vi "Module A.vi"(8 "Error In":errorcluster) -> (0 "Error Out":errorcluster)   [LabVIEW 2024]
panel:
  in  "Stop":bool
  out "Elapsed Time":dbl format="%.3f seconds"
  out "Loop iteration":i32
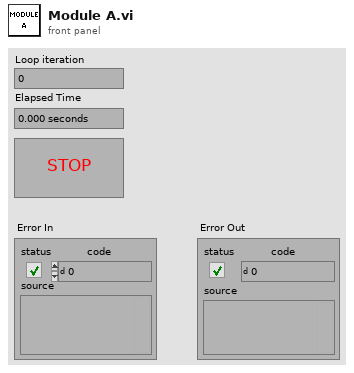
[diagram p1: front panel]
types:
  T1 = enum32{"Invalid", "Standard", "Closed", "Hidden", "Minimized", "Maximized"}
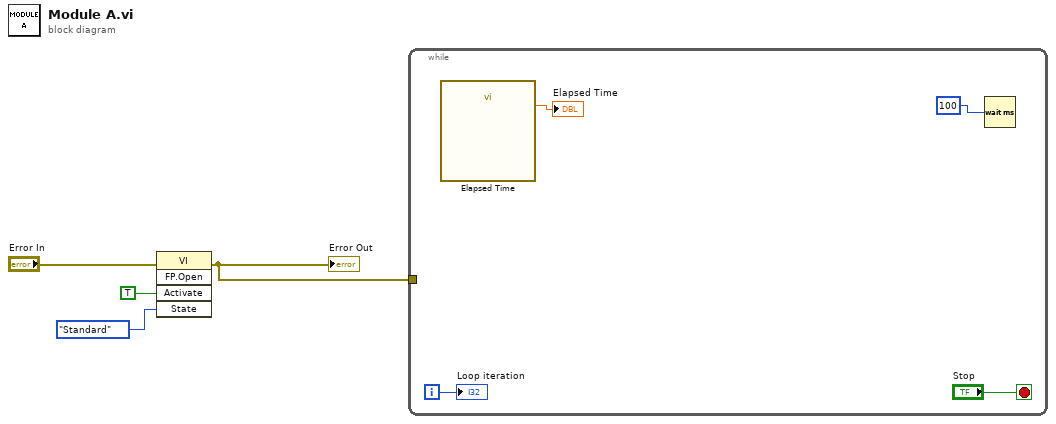
[diagram p0: block diagram]
diagram:
  n1 = invoke class="VI" method="FP.Open"(error in="Error In", "Activate"=TRUE ("Activate?"), "State"=T1."Standard" ("Front Panel Window:State")) -> (error out=w3:errorcluster)  [unwired: 2 in, 4 out]
  "Error Out" <- w3
  n2 = while {
    tunnel: w3 -> [_]
    i -> [w7]
    stop <- "Stop" stop-if-true
    n3 = call "Elapsed Time"() -> ("Elapsed Time (s)"=→"Elapsed Time":dbl)  [unwired: 12 in, 7 out]
    n4 = Wait (ms)(milliseconds to wait=u32 100) -> ()  [unwired: 1 out]
    "Loop iteration" <- w7
  }
